vi "Event FGV.vi"(8 "error in (no error)":errorcluster, 11 "State":T1) -> (0 "error out":errorcluster, 3 "Stop All":refnum<user-event>)   [LabVIEW 2014]
uses:
  Event State.ctl
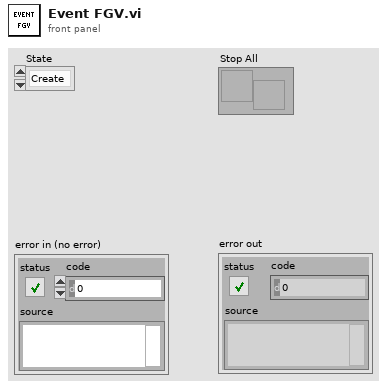
[diagram p1: front panel]
types:
  T1 = typedef "Event State.ctl" = enum16{"Create", "Get", "Destroy"}
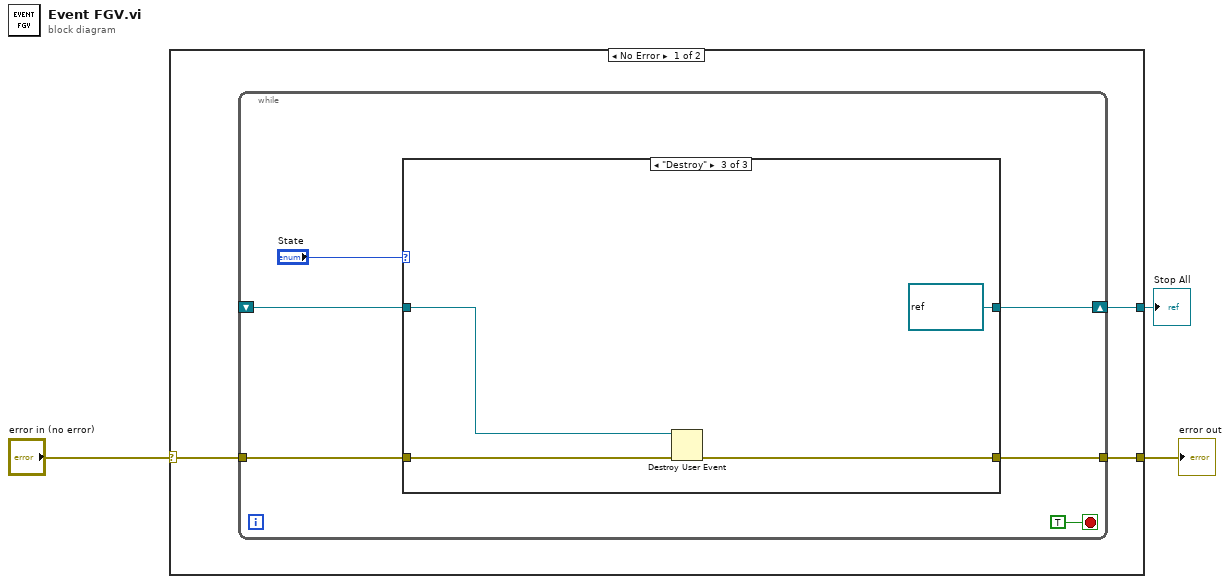
[diagram p0: block diagram]
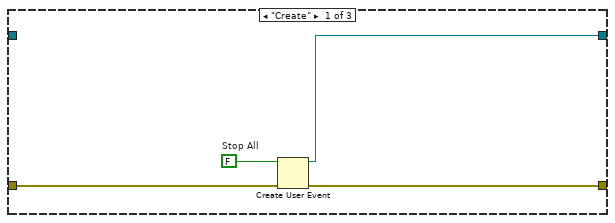
[diagram p2: hidden frame]
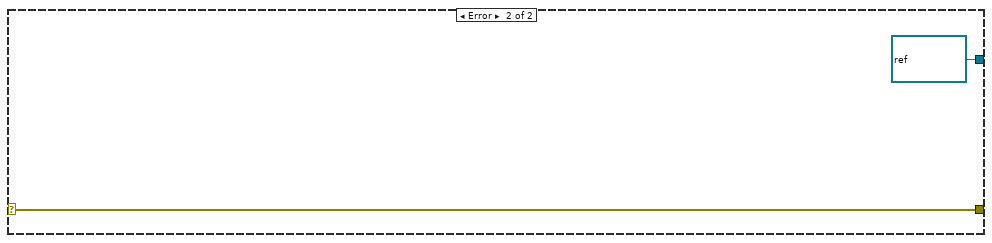
[diagram p4: hidden frame]
diagram:
  n1 = case shown="No Error" "error in (no error)" {
    selector: "error in (no error)" -> [w6 w23]
    tunnel: [w5 w23] -> w2
    tunnel: [w4 refnum<user-event> refnum ("Stop All")] -> w1
    frame No Error {
      n2 = while {
        tunnel: w6 -> [w11]
        tunnel: [w9] -> w5
        shift-right: [w8] -> w4
        shift-left: _ -> [w7]
        stop <- TRUE stop-if-true
        n3 = case shown="\"Destroy\"" "State" {
          tunnel: w11 -> [w16 w17 w22]
          tunnel: [w15 w17 w21] -> w9
          tunnel: [w13 w18 refnum<user-event> refnum ("Stop All")] -> w8
          tunnel: w7 -> [_ w18 w20]
          frame "Create" {
            w14 = FALSE  # Stop All
            n4 = Create User Event(user event datatype=w14, error in=w16) -> (user event=w13:refnum<user-event>, error out=w15:errorcluster)
          }
          frame "Get", Default {
          }
          frame "Destroy" {
            n5 = Destroy User Event(user event=w20, error in=w22) -> (error out=w21:errorcluster)
          }
        }
      }
    }
    frame Error {
    }
  }
  "error out" <- w2
  "Stop All" <- w1
